vi "MB lesen.vi"(0 "TCP Refnum":refnum<k5>, 3 "Adresse":u16[](array[numeric]), 7 "error in":errorcluster, 13 "Aktion":T1) -> (20 "TCP Refnum":refnum<k5>, 21 "Exception Code":u8, 22 "Holding Registers":u16[](array[numeric]), 23 "Input Registers":u16[](array[numeric]), 24 "Discrete Inputs":bool[](array[boolean]), 25 "Coils":bool[](array[boolean]), 27 "error out":errorcluster)   [LabVIEW 2020, in "ABB-EL3000.lvlib" / "Allgemeine VI.lvlib"]
uses:
  Allgemeine VI.lvlib
  Aktion Modbus lesen.ctl
  <userlib>/NI Modbus.llb/MB Ethernet Master Query Read Coils (poly).vi
  <userlib>/NI Modbus.llb/MB Ethernet Master Query Read Discrete Inputs (poly).vi
  <userlib>/NI Modbus.llb/MB Ethernet Master Query Read Input Registers (poly).vi
  <userlib>/NI Modbus.llb/MB Ethernet Master Query Read Holding Registers (poly).vi
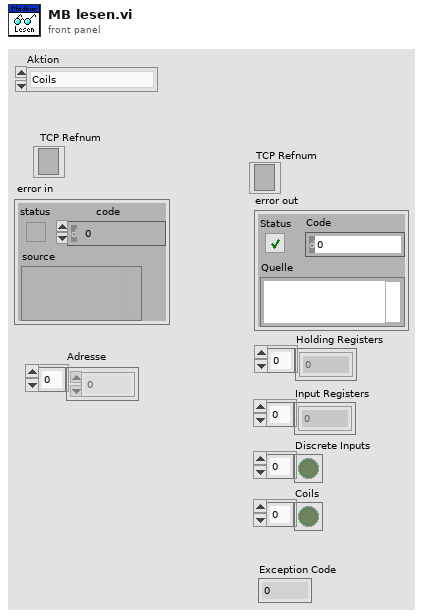
[diagram p1: front panel]
types:
  T1 = typedef "ABB-EL3000.lvlib/Allgemeine VI.lvlib/Aktion Modbus lesen.ctl" = enum16{"Coils", "Discrete Inputs", "Input Register", "Holding Register"}
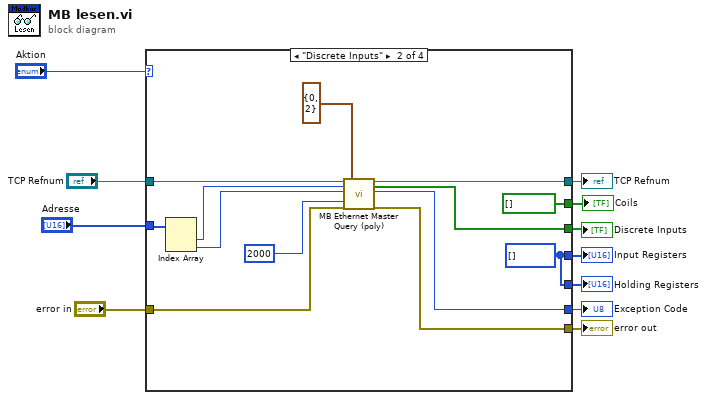
[diagram p0: block diagram]
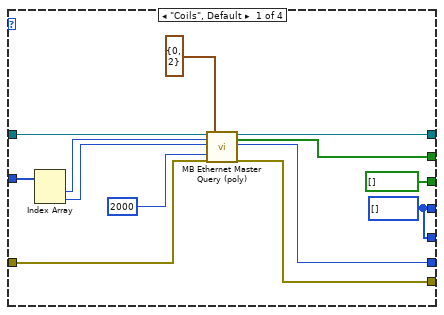
[diagram p2: hidden frame]
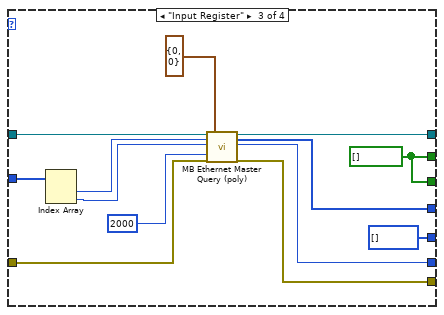
[diagram p3: hidden frame]
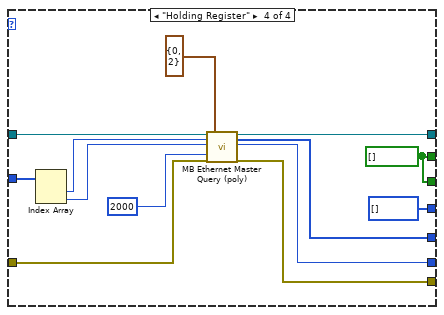
[diagram p4: hidden frame]
diagram:
  n1 = case shown="\"Discrete Inputs\"" "Aktion" {
    tunnel: "TCP Refnum" -> [w24 w37 w50 w63]
    tunnel: [w21 w34 w47 w60] -> w9
    tunnel: [w20 bool[] [] ("Coils") w42 w56] -> w5
    tunnel: [w19 w33 w46 w59] -> w6
    tunnel: "error in" -> [w18 w32 w45 w58]
    tunnel: [w17 w31 w44 w57] -> w7
    tunnel: [bool[] [] ("Coils") w30 w42 w56] -> w4
    tunnel: [w15 w28 w43 u16[] [] ("Input Registers")] -> w3
    tunnel: [w15 w28 u16[] [] ("Holding Registers") w54] -> w2
    tunnel: "Adresse" -> [w14 w27 w40 w53]
    frame "Coils", Default {
      w15 = u16[] [] ("Input Registers")
      n2 = Index Array(array=w14) -> (element #1=w13:u16, element #2=w12:u16)  [unwired: 2 in]
      n3 = call-poly <userlib>:"MB Ethernet Master Query (poly).vi"("TCP Connection Refnum in"=w24, "Starting Address"=w13, "Quantity"=w12, "Timeout"=2000, "error in"=w18, "MBAP Header"=cluster{"Transaction ID":u16, "Unit ID":u8} {"Transaction ID"=0, "Unit ID"=2}) -> ("TCP Connection Refnum (dup)"=w21:refnum<k5>, "Coils"=w20:bool[], "Exception Code"=w19:u8, "error out"=w17:errorcluster)  [unwired: 10 in]
    }
    frame "Discrete Inputs" {
      w28 = u16[] [] ("Input Registers")
      n4 = Index Array(array=w27) -> (element #1=w26:u16, element #2=w25:u16)  [unwired: 2 in]
      n5 = call-poly <userlib>:"MB Ethernet Master Query (poly).vi"("TCP Connection Refnum in"=w37, "Starting Address"=w26, "Quantity"=w25, "Timeout"=2000, "error in"=w32, "MBAP Header"=cluster{"Transaction ID":u16, "Unit ID":u8} {"Transaction ID"=0, "Unit ID"=2}) -> ("TCP Connection Refnum (dup)"=w34:refnum<k5>, "Discrete Inputs"=w30:bool[], "Exception Code"=w33:u8, "error out"=w31:errorcluster)  [unwired: 10 in]
    }
    frame "Input Register" {
      w42 = bool[] [] ("Coils")
      n6 = Index Array(array=w40) -> (element #1=w39:u16, element #2=w38:u16)  [unwired: 2 in]
      n7 = call-poly <userlib>:"MB Ethernet Master Query (poly).vi"("TCP Connection Refnum in"=w50, "Starting Address"=w39, "Quantity"=w38, "Timeout"=2000, "error in"=w45, "MBAP Header"=cluster{"Transaction ID":u16, "Unit ID":u8} {"Transaction ID"=0, "Unit ID"=0}) -> ("TCP Connection Refnum (dup)"=w47:refnum<k5>, "Input Registers"=w43:u16[], "Exception Code"=w46:u8, "error out"=w44:errorcluster)  [unwired: 10 in]
    }
    frame "Holding Register" {
      w56 = bool[] [] ("Coils")
      n8 = Index Array(array=w53) -> (element #1=w52:u16, element #2=w51:u16)  [unwired: 2 in]
      n9 = call-poly <userlib>:"MB Ethernet Master Query (poly).vi"("TCP Connection Refnum in"=w63, "Starting Address"=w52, "Quantity"=w51, "Timeout"=2000, "error in"=w58, "MBAP Header"=cluster{"Transaction ID":u16, "Unit ID":u8} {"Transaction ID"=0, "Unit ID"=2}) -> ("TCP Connection Refnum (dup)"=w60:refnum<k5>, "Holding Registers"=w54:u16[], "Exception Code"=w59:u8, "error out"=w57:errorcluster)  [unwired: 10 in]
    }
  }
  "TCP Refnum" <- w9
  "error out" <- w7
  "Exception Code" <- w6
  "Coils" <- w5
  "Discrete Inputs" <- w4
  "Input Registers" <- w3
  "Holding Registers" <- w2
